vi "Check If Client Connection Valid.vi"(7 "return error if invalid (T)":bool=TRUE, 8 "error in":errorcluster, 11 "connection ID in":T1) -> (0 "error out":errorcluster, 2 "valid?":bool, 3 "connection ID out":T1)   [LabVIEW 2010, in "NI_CCC.lvlib"]
uses:
  NI_CCC.lvlib
  Connection ID.ctl
  <vilib>/NI/STM/TCP/TCP Connection Info.ctl
  <vilib>/NI/STM/SubVIs/MetaDataElement.ctl
  Tag Configuration.ctl
  <vilib>/NI/Current Value Table/Type Defs/Data Types.ctl
  Tag Direction.ctl
  <vilib>/NI/Current Value Table/Current Value Table.lvlib
  <vilib>/NI/STM/NI STM.lvlib
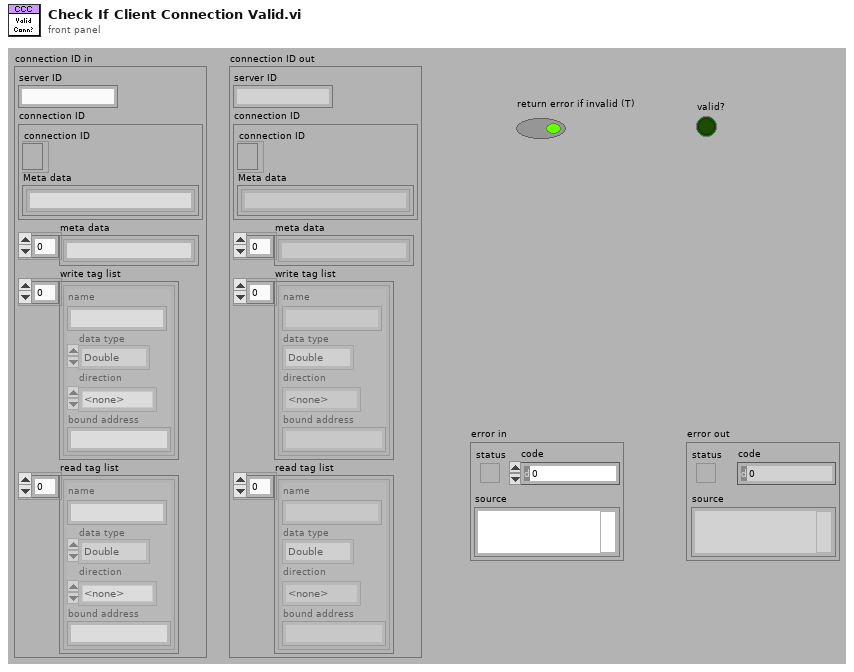
[diagram p1: front panel]
types:
  T1 = typedef "NI_CCC.lvlib/Connection ID.ctl" = cluster{"server ID":string, "connection ID":T2, "meta data":T3[], "write tag list":T4[], "read tag list":T4[]}
  T2 = typedef "NI STM.lvlib/TCP Connection Info.ctl" = cluster{"connection ID":refnum<k5>, "Meta data":T3[]}
  T3 = typedef "NI STM.lvlib/MetaDataElement.ctl" = string
  T4 = typedef "NI_CCC.lvlib/Tag Configuration.ctl" = cluster{"name":string, "data type":T5, "direction":T6, "bound address":string}
  T5 = typedef "Current Value Table.lvlib/Data Types.ctl" = enum16{"Double", "Single", "I64", "I32", "I16", "I8", "U64", "U32", "U16", "U8", "String", "Boolean", "Array of U8", "Array of U16", "Array of U32", "Array of U64", "Array of I64", "Array of I32", "Array of I16", "Array of I8", "Array of Double", "Array of Single", "Array of Boolean", "Array of String"}
  T6 = typedef "NI_CCC.lvlib/Tag Direction.ctl" = enum32{"<none>", "Read", "Write"}
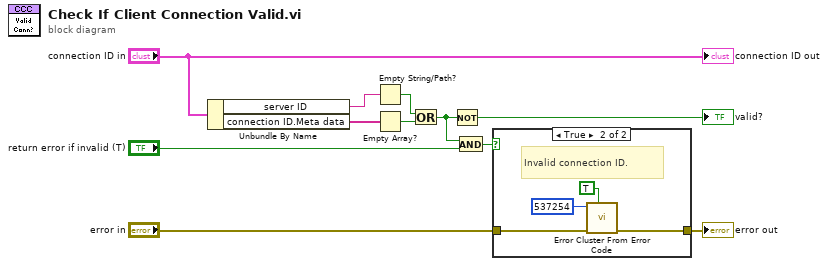
[diagram p0: block diagram]
diagram:
  n1 = Unbundle By Name("connection ID in") -> ("server ID"=w10:string, "connection ID.Meta data"=w8:T3[])
  n2 = Empty String/Path?(string/path=w10) -> (empty?=w7:bool)
  n3 = Empty Array?(array=w8) -> (empty?=w6:bool)
  n4 = Or(x=w7, y=w6) -> (x .or. y?=w5:bool)
  n5 = Not(x=w5) -> (.not. x?=→"valid?":bool)
  n6 = And(x=w5, y="return error if invalid (T)") -> (x .and. y?=w3:bool)
  n7 = case shown="True" w3 {
    tunnel: "error in" -> [w12 w14]
    tunnel: [w12 w13] -> w1
    frame False {
    }
    frame True {
      # "Invalid connection ID."
      n8 = call <vilib>:"Error Cluster From Error Code.vi"("show call chain? (False)"=TRUE, "error in (no error)"=w14, "error code (0)"=537254) -> ("error out"=w13:errorcluster)  [unwired: 6 out]
    }
  }
  "error out" <- w1
  "connection ID out" <- "connection ID in"
